vi "Configure Measurement Parameter.vi"(6 "Measurement Type (0: S11)":i32(ring) items=["S11", "S12", "S21", "S22", "A", "B", "R1", "R2", "A/B", "B/A"], 7 "Mode (0: Create)":u16(ring) items=["Create", "Delete", "Select"], 8 "Error In (no error)":errorcluster, 9 "Measurement Name (MY_MEAS)":string="MY_MEAS", 10 "Channel (1)":i32=1, 11 "VISA Resource Name":refnum<visa-resource-name>) -> (0 "Error Out":errorcluster, 3 "VISA Resource Name Out":refnum<visa-resource-name>)   [LabVIEW 2018, in "Agilent PNA Series.lvlib"]
doc: "This VI creates, deletes or selects a measurement parameter for the selected channel. \n\nNote: This VI does not cause the parameter to be displayed. Use the \"AGPNA Create Display Trace.vi\" to display the measurement parameter.\n\nThe Select mode is not required for normal driver operation. It is provided for convenience."
uses:
  Agilent PNA Series.lvlib
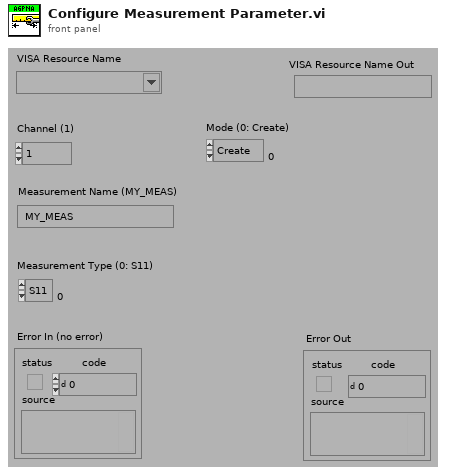
[diagram p1: front panel]
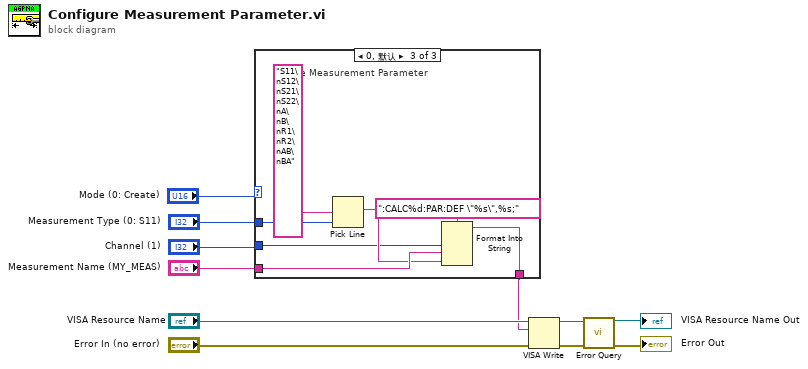
[diagram p0: block diagram]
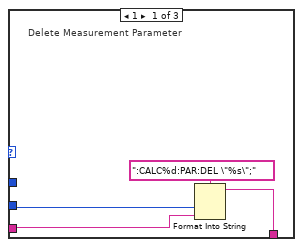
[diagram p2: hidden frame]
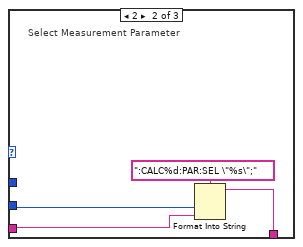
[diagram p3: hidden frame]
diagram:
  n1 = case shown="0, 默认" "Mode (0: Create)" {
    tunnel: "Channel (1)" -> [w14 w18 w20]
    tunnel: "Measurement Name (MY_MEAS)" -> [w13 w17 w25]
    tunnel: "Measurement Type (0: S11)" -> [_ _ w23]
    tunnel: [w12 w16 w21] -> w5
    frame 1 {
      # "Delete Measurement Parameter"
      n2 = Format Into String(format string=":CALC%d:PAR:DEL \"%s\";", w14, w13) -> (resulting string=w12:string)  [unwired: 2 in, 1 out]
    }
    frame 2 {
      # "Select Measurement Parameter"
      n3 = Format Into String(format string=":CALC%d:PAR:SEL \"%s\";", w18, w17) -> (resulting string=w16:string)  [unwired: 2 in, 1 out]
    }
    frame 0, Default {
      # "Create Measurement Parameter"
      n4 = Pick Line(multi-line string="S11\nS12\nS21\nS22\nA\nB\nR1\nR2\nAB\nBA", line index=w23) -> (output string=w22:string)  [unwired: 1 in]
      n5 = Format Into String(format string=":CALC%d:PAR:DEF \"%s\",%s;", w20, w25, w22) -> (resulting string=w21:string)  [unwired: 2 in, 1 out]
    }
  }
  n6 = VISA Write(VISA resource name="VISA Resource Name", write buffer=w5, error in (no error)="Error In (no error)") -> (VISA resource name out=w4:refnum<visa-resource-name>, error out=w3:errorcluster)  [unwired: 1 out]
  n7 = call "Error Query.vi"("VISA Resource Name"=w4, "error in (no error)"=w3) -> ("VISA Resource Name Out"=→"VISA Resource Name Out":refnum<visa-resource-name>, "error out"=→"Error Out":errorcluster)  [unwired: 10 in, 2 out]
